vi "save coor order.vi"(10 "Save Coordinates":T1(array[cluster])=[{"ROI name"="", "pixel coordinates"={"x"=0, "y"=0}}, {"ROI name"="", "pixel coordinates"={"x"=0, "y"=0}}, {"ROI name"="", "pixel coordinates"={"x"=0, "y"=0}}], 11 "Stm ID":string[](array[string])=["1", "4", "2", "6", "3", "5"]) -> (3 "New ROI":string[](array[string]))   [LabVIEW 2012]
uses:
  save ROI.vi
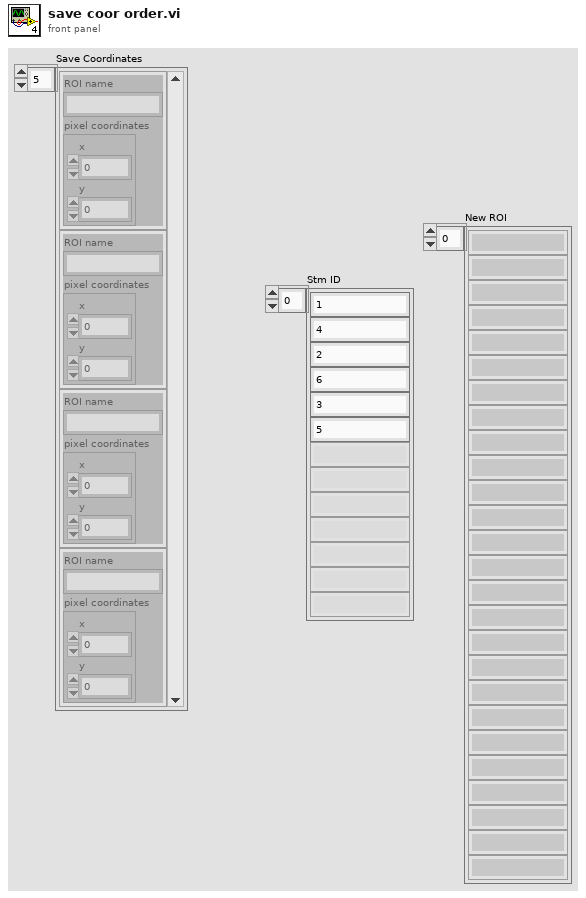
[diagram p1: front panel]
types:
  T1 = cluster{"ROI name":string, "pixel coordinates":cluster{"x":i32, "y":i32}}[]
  T2 = cluster{"ROI name":string, "pixel coordinates":cluster{"x":i32, "y":i32}}
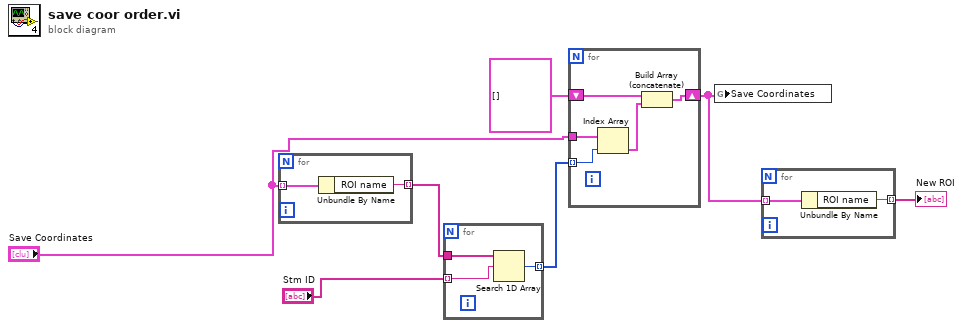
[diagram p0: block diagram]
diagram:
  n1 = for {
    tunnel: "Save Coordinates" -> [w9] mode=indexing
    tunnel: [w8] -> w7 mode=indexing
    n2 = Unbundle By Name(w9) -> ("ROI name"=w8:string)
  }
  n3 = for {
    tunnel: "Stm ID" -> [w11] mode=indexing
    tunnel: w7 -> [w12]
    tunnel: [w10] -> w5 mode=indexing
    n4 = Search 1D Array(1D array=w12, element=w11) -> (index of element=w10:i32)  [unwired: 1 in]
  }
  n5 = for {
    tunnel: w5 -> [w16] mode=indexing
    tunnel: "Save Coordinates" -> [w17]
    shift-right: [w13] -> w3
    shift-left: T1 [] -> [w14]
    n6 = Index Array(array=w17, index=w16) -> (element=w15:T2)
    n7 = Build Array (concatenate)(w14, w15) -> (w13:T1)
  }
  n8 = global write "save ROI.vi" "Save Coordinates"(w3) -> ()
  n9 = for {
    tunnel: w3 -> [w19] mode=indexing
    tunnel: [w18] -> w2 mode=indexing
    n10 = Unbundle By Name(w19) -> ("ROI name"=w18:string)
  }
  "New ROI" <- w2
